vi "ReadLastOF.vi"(8 "errin":errorcluster) -> (0 "errout":errorcluster, 1 "VISA HITECH":string, 2 "VISA Auto":string caption="VISA", 3 "OF":string)   [LabVIEW 2020]
uses:
  <vilib>/Utility/config.llb/Read Key (String).vi
  <vilib>/Utility/config.llb/NI_LVConfig.lvlib
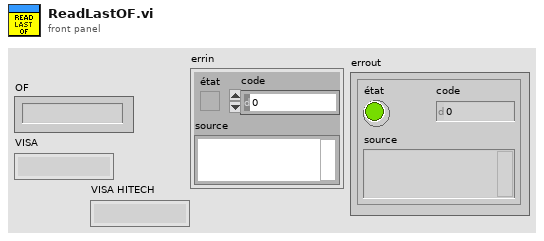
[diagram p1: front panel]
types:
  T1 = typedef "NI_LVConfig.lvlib/Config Data RefNum.ctl" = refnum<k1>
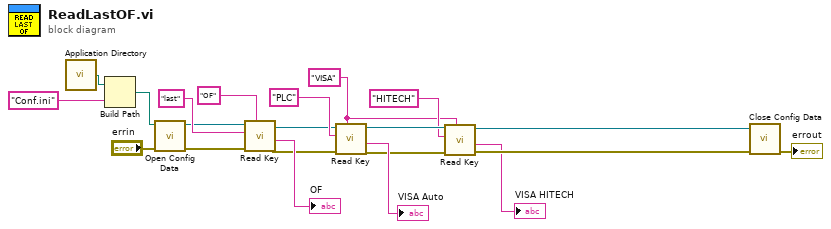
[diagram p0: block diagram]
diagram:
  w1 = "VISA" ("section")
  n1 = call <vilib>:"Application Directory.vi"() -> ("Application Directory"=w15:path)
  n2 = Build Path ("Composer un chemin")(base path=w15, name or relative path="Conf.ini") -> (appended path=w17:path)
  n3 = call <vilib>:"Open Config Data.vi"("error in (no error)"="errin", "configuration file path"=w17) -> ("error out"=w13:errorcluster, "refnum"=w18:T1)  [unwired: 7 in, 1 out]
  n4 = call-poly <vilib>:"Read Key.vi"("section"="OF", "error in (no error)"=w13, "key"="last", "refnum"=w18) -> ("error out"=w11:errorcluster, "value"=→"OF":string, "refnum out"=w8:T1)  [unwired: 4 in, 1 out]
  n5 = call-poly <vilib>:"Read Key.vi"("section"=w1, "error in (no error)"=w11, "key"="PLC" ("section"), "refnum"=w8) -> ("error out"=w4:errorcluster, "value"=→"VISA Auto":string, "refnum out"=w7:T1)  [unwired: 4 in, 1 out]
  n6 = call-poly <vilib>:"Read Key.vi"("section"=w1, "error in (no error)"=w4, "key"="HITECH" ("section"), "refnum"=w7) -> ("error out"=w5:errorcluster, "value"=→"VISA HITECH":string, "refnum out"=w6:T1)  [unwired: 4 in, 1 out]
  n7 = call <vilib>:"Close Config Data.vi"("error in (no error)"=w5, "refnum"=w6) -> ("error out"=→"errout":errorcluster)  [unwired: 8 in, 1 out]
